vi "Add Menu Measurement.vi"(8 "error in (no error)":errorcluster, 10 "Name":string, 11 "Common Measurements Interface in":refnum<class "Common Measurements Interface.lvclass">) -> (0 "error out":errorcluster, 3 "Common Measurements Interface out":refnum<class "Common Measurements Interface.lvclass">)   [LabVIEW 2015, in "Common Measurements Interface.lvclass"]
uses:
  Common Measurements Interface.lvclass
  Common Measurements Interface.lvclass/Common Measurements Interface.ctl
  Queued Listbox/Queued Listbox.xctl
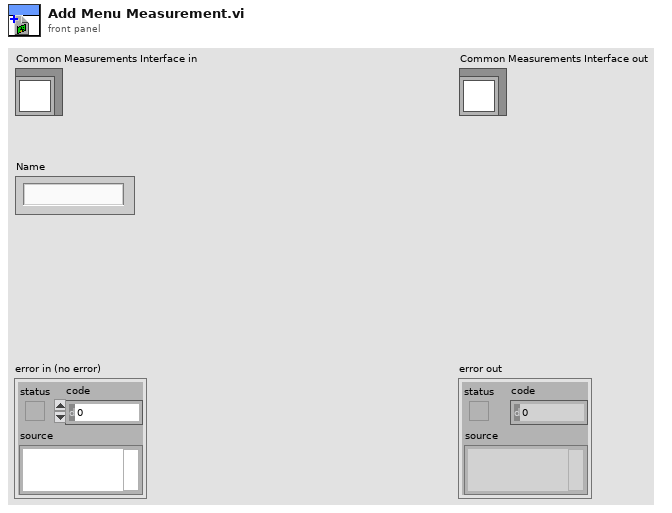
[diagram p1: front panel]
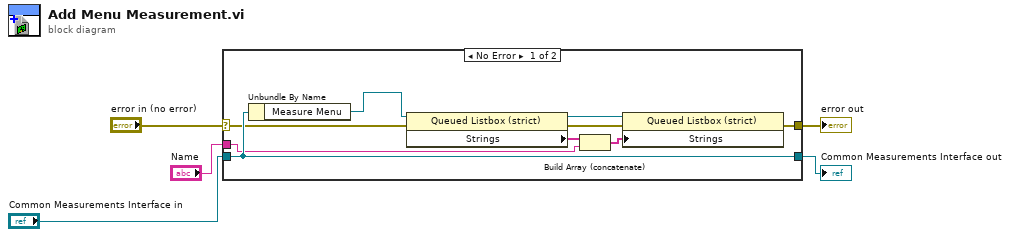
[diagram p0: block diagram]
diagram:
  n1 = case shown="No Error" "error in (no error)" {
    selector: "error in (no error)" -> [w10 w16]
    tunnel: [w7 w16] -> w4
    tunnel: [w14 w15] -> w2
    tunnel: "Common Measurements Interface in" -> [w14 w15]
    tunnel: "Name" -> [w11 _]
    frame No Error {
      n2 = Unbundle By Name(w14) -> ("Measure Menu"=w6:refnum<vi>)
      n3 = property class="Queued Listbox (strict)"(reference=w6, error in=w10) -> (reference out=w13:refnum<vi>, error out=w9:errorcluster, "Strings"=w12:string[])
      n4 = Build Array (concatenate)(w12, w11) -> (w8:string[])
      n5 = property class="Queued Listbox (strict)"(reference=w13, error in=w9, "Strings"=w8) -> (error out=w7:errorcluster)  [unwired: 1 out]
    }
    frame Error {
    }
  }
  "error out" <- w4
  "Common Measurements Interface out" <- w2
